vi "Read ScanCode.vi"(8 "error in (no error)":errorcluster, 11 "ControlKeyDownMsg in":refnum<class "VIKeyDownMsg.lvclass">) -> (0 "error out":errorcluster, 2 "ScanCode":i16, 3 "ControlKeyDownMsg out":refnum<class "VIKeyDownMsg.lvclass">)   [LabVIEW 2020, in "MVA Framework.lvlib" / "ActorEvents.lvlib" / "VIKeyDownMsg.lvclass"]
uses:
  VIKeyDownMsg.lvclass
  VIKeyDownMsg.lvclass/VIKeyDownMsg.ctl
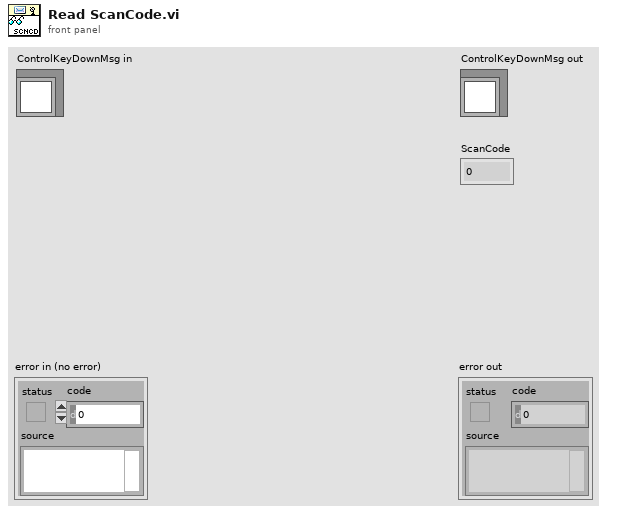
[diagram p1: front panel]
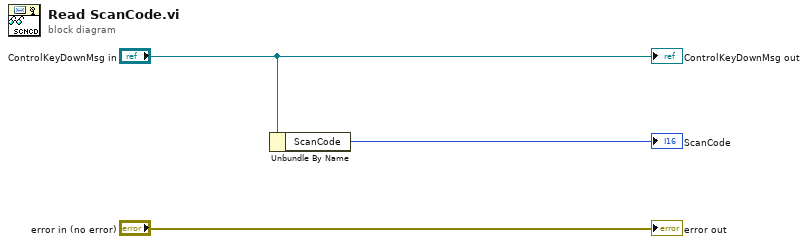
[diagram p0: block diagram]
diagram:
  n1 = Unbundle By Name("ControlKeyDownMsg in") -> ("ScanCode"=→"ScanCode":i16)
  "error out" <- "error in (no error)"
  "ControlKeyDownMsg out" <- "ControlKeyDownMsg in"
